vi "Resample to new X.vi"(5 "offset length":i32=990000, 6 "Integrate Bdot":bool, 7 "Bdot calibration":dbl=2506.0, 8 "Error In":errorcluster, 10 "Signal":waveform(dbl)[](array[waveform]), 11 "X-axis file":path) -> (0 "Error Out":errorcluster, 1 "XY Graph":cluster{dbl[], "Y":dbl[]}[](graph), 2 "Resampled Signal":waveform(dbl)[](array[waveform]), 3 "X-axis file out":path)   [LabVIEW 2015]
uses:
  <vilib>/Analysis/NI_AALPro.lvlib
panel:
  in  "Bdot channel":string="Field_fixed"
  in  "Filed tiime shift":dbl format="%#_6p"
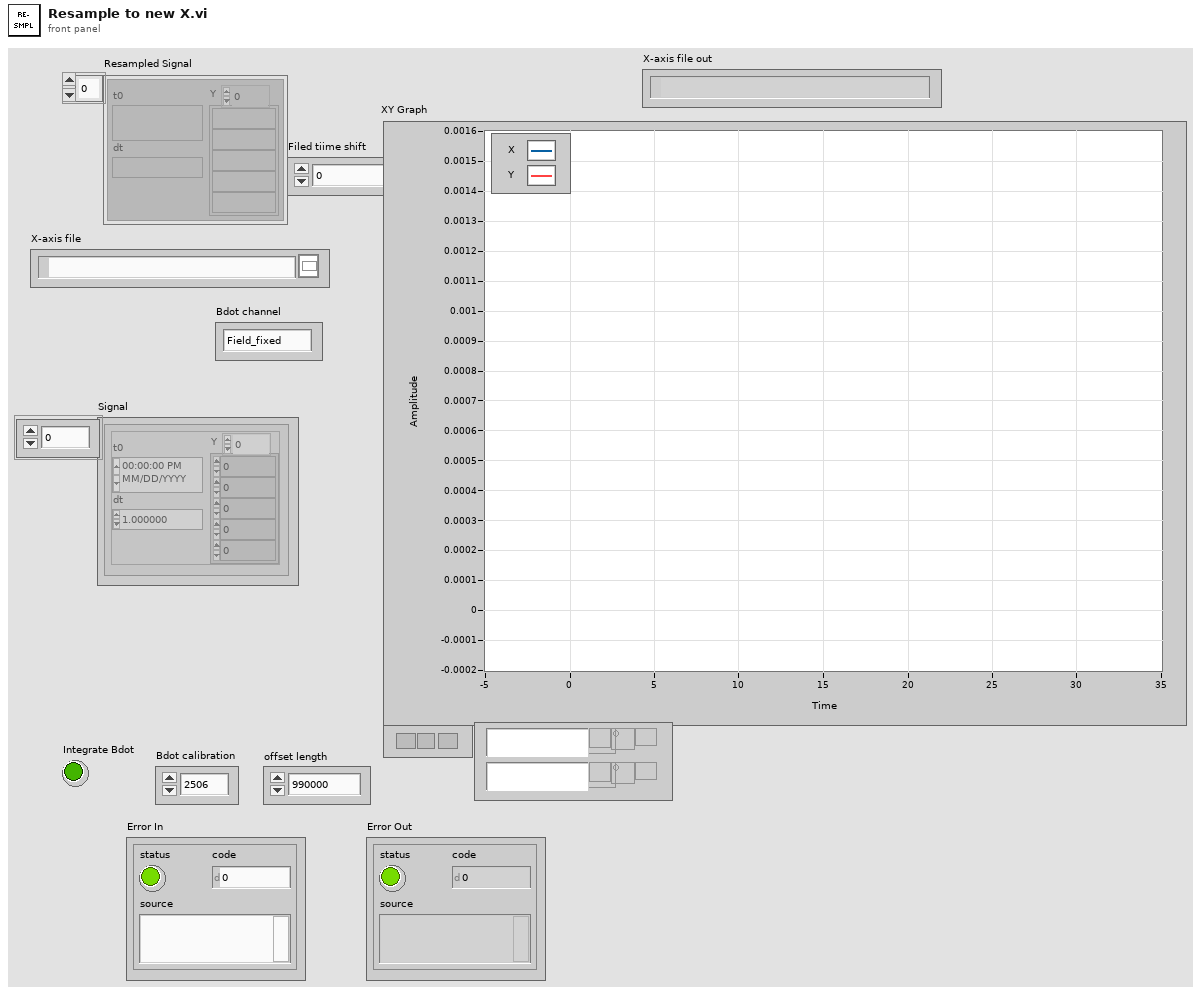
[diagram p1: front panel]
types:
  T1 = enum16{"open", "open or create", "create or replace", "create", "open (read-only)"}
  T2 = cluster{"Waveform":waveform(dbl), "Waveform":waveform(dbl)}
  T3 = cluster{"Waveform":waveform(dbl), "Waveform":waveform(dbl)}[]
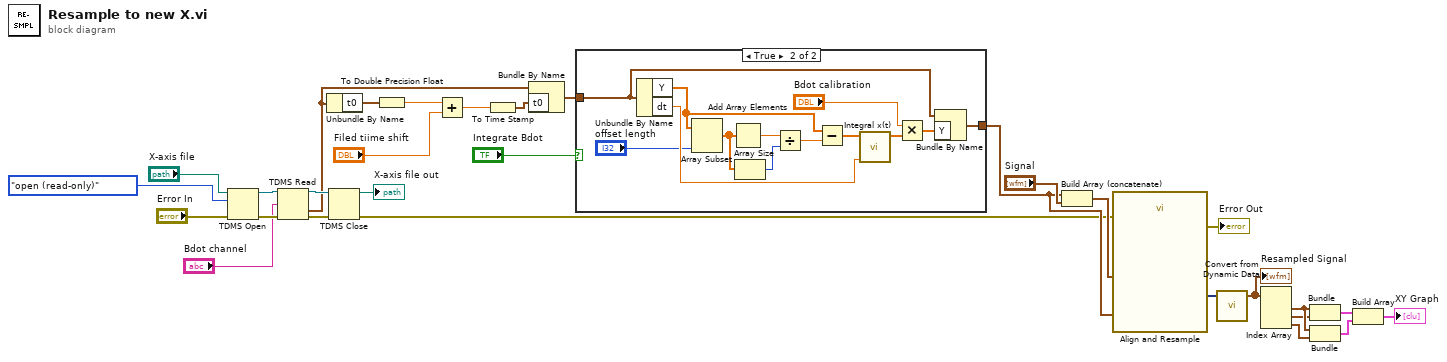
[diagram p0: block diagram]
diagram:
  n1 = TDMS Open(8:"Error In", 10:T1."open (read-only)" ("operation (0:open)"), 11:"X-axis file") -> (0:w25:errorcluster, 3:w24:refnum<k34>)  [unwired: 4 in]
  n2 = TDMS Read(0:w24, 7:"Bdot channel", 11:w25) -> (4:w21:refnum<k34>, 10:w3:waveform(dbl), 15:w22:errorcluster)  [unwired: 5 in, 3 out]
  n3 = Unbundle By Name(w3) -> ("t0"=w8:timestamp)
  n4 = TDMS Close(8:w22, 11:w21) -> (0:w9:errorcluster, 3:→"X-axis file out":path)
  n5 = To Double Precision Float(number=w8) -> (double precision float=w7:dbl)
  n6 = Add(x=w7, y="Filed tiime shift") -> (x+y=w5:dbl)
  n7 = To Time Stamp(1:w5) -> (0:w4:timestamp)
  n8 = Bundle By Name(cluster=w3, "t0"=w4) -> (w2:waveform(dbl))
  n9 = case shown="True" "Integrate Bdot" {
    tunnel: w2 -> [w31 w34]
    tunnel: [w31 w32] -> w19
    frame False {
    }
    frame True {
      n10 = Unbundle By Name(w34) -> ("Y"=w37:dbl[], "dt"=w44:dbl)
      n11 = Array Subset(array=w37, length="offset length") -> (w41:dbl[])  [unwired: 1 in]
      n12 = Add Array Elements(numeric array=w41) -> (sum=w40:dbl)
      n13 = Array Size(array=w41) -> (size(s)=w39:i32)
      n14 = Divide(x=w40, y=w39) -> (x/y=w36:dbl)
      n15 = Subtract(x=w37, y=w36) -> (x-y=w38:dbl[])
      n16 = call <vilib>:"Integral x(t).vi"("dt"=w44, "X"=w38) -> ("Integral X"=w43:dbl[])  [unwired: 8 in, 1 out]
      n17 = Multiply(x="Bdot calibration", y=w43) -> (x*y=w33:dbl[])
      n18 = Bundle By Name(cluster=w34, "Y"=w33) -> (w32:waveform(dbl))
    }
  }
  n19 = Build Array (concatenate)(w19, "Signal") -> (w13:waveform(dbl)[])
  n20 = call "Align and Resample"("Reference Signal"=w19, "error in (no error)"=w9, "Signals"=w13) -> ("error out"=→"Error Out":errorcluster, "Resampled Signals"=w18:dynamicdata)  [unwired: 6 in, 1 out]
  n21 = call "Convert from Dynamic Data"("Dynamic Data Type"=w18) -> ("Array of Waveform"=w10:waveform(dbl)[])  [unwired: 3 in]
  "Resampled Signal" <- w10
  n22 = Index Array(array=w10) -> (element #1=w17:waveform(dbl), element #2=w12:waveform(dbl), element #3=w11:waveform(dbl))  [unwired: 3 in]
  n23 = Bundle("Waveform"=w17, "Waveform"=w12) -> (w16:T2)  [unwired: 1 in]
  n24 = Bundle("Waveform"=w17, "Waveform"=w11) -> (w15:T2)  [unwired: 1 in]
  n25 = Build Array(w16, w15) -> (→"XY Graph":T3)
